vi "RTR.vi"(0 "System no.":i32=1 min=1 max=4 step=1, 2 "Table rate":i32=1, 5 "error in":errorcluster) -> (14 "Controller error":bool, 19 "error out":errorcluster)   [LabVIEW 2020]
doc: "This VI sets the table rate and queries ERR?. The table rate is the number of servo-loop cycles to be used in data recording operations. Settings larger than 1 make it possible to cover longer time periods with a limited number of points. Controller error is TRUE if selected system report error code not equal to zero. \n\nC-887, F-206, M-8X0: Only for GCS syntax version = GCS 2.0 or higher (Check with CSV?.vi. If CSV?.vi is not supported, syntax version is GCS 1.0)."
panel:
  # "This vi sets the table rate and queries ERR?."
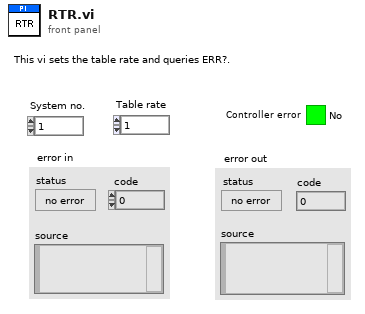
[diagram p1: front panel]
types:
  T1 = enum16{"Disable error check", "Force error check", "Use global settings"}
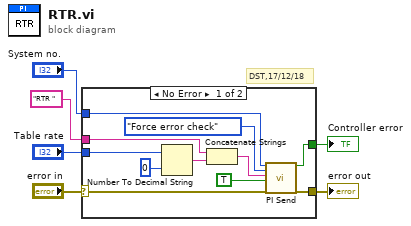
[diagram p0: block diagram]
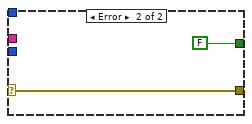
[diagram p2: hidden frame]
diagram:
  # "DST,17/12/18"
  n1 = case shown="No Error" "error in" {
    selector: "error in" -> [w10 w18]
    tunnel: [w8 w18] -> w6
    tunnel: "RTR " -> [w17 _]
    tunnel: "System no." -> [w15 _]
    tunnel: [w9 FALSE ("Controller error")] -> w3
    tunnel: "Table rate" -> [w13 _]
    frame No Error {
      n2 = Number To Decimal String(number=w13, width (-)=i16 0) -> (decimal integer string=w11:string)
      n3 = Concatenate Strings(w17, w11) -> (w14:string)
      n4 = call "PI Send.vi"("System no."=w15, "Error check settings"=T1."Force error check", "String to send"=w14, "Attach termination char.?"=TRUE ("Attach Linefeed?"), "error in"=w10) -> ("Controller error"=w9:bool, "error out"=w8:errorcluster)  [unwired: 1 in, 12 out]
    }
    frame Error {
    }
  }
  "error out" <- w6
  "Controller error" <- w3
